vi "MTM2_putSample_ilcData.vi"(8 "error in (no error)":errorcluster, 11 "ilcData_Ctl":T1={"private_rcvStamp"=0.0, "status[78]"=[0, 0, 0, 0, 0, 0, 0, 0, 0, 0, 0, 0, 0, 0, 0, 0, 0, 0, 0, 0, 0, 0, 0, 0, 0, 0, 0, 0, 0, 0, 0, 0, 0, 0, 0, 0, 0, 0, 0, 0, 0, 0, 0, 0, 0, 0, 0, 0, 0, 0, 0, 0, 0, 0, 0, 0, 0, 0, 0, 0, 0, 0, 0, 0, 0, 0, 0, 0, 0, 0, 0, 0, 0, 0, 0, 0, 0, 0]}) -> (0 "error out":errorcluster, 2 "function return":i32, 3 "ilcData_Ctl out":T1)   [LabVIEW 2018, in "SALLV_MTM2.lvlib"]
doc: "int MTM2_shm_putSample_ilcDataLV(MTM2_ilcDataLV *ilcData_Ctl );"
uses:
  DataTypes/ilcData.ctl
  SALLV_MTM2.lvlib
  SALLV_MTM2.so
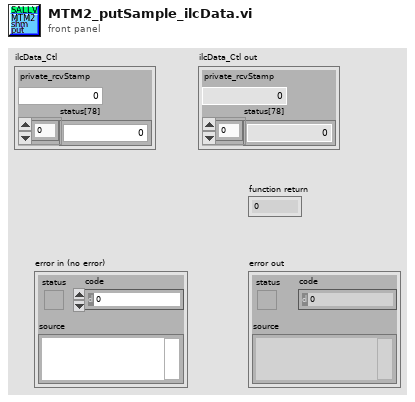
[diagram p1: front panel]
types:
  T1 = typedef "SALLV_MTM2.lvlib/ilcData.ctl" = cluster{"private_rcvStamp":dbl, "status[78]":u16[]}
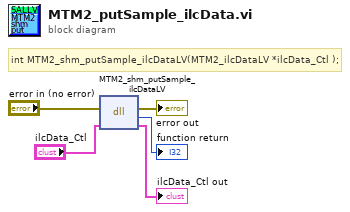
[diagram p0: block diagram]
diagram:
  # "int MTM2_shm_putSample_ilcDataLV(MTM2_ilcDataLV *ilcData_Ctl );"
  n1 = dll-call lib="home/ttsai/Documents/salLabviewApi/SALLV_MTM2/SALLV_MTM2.*" fn="MTM2_shm_putSample_ilcDataLV"(error in="error in (no error)", "ilcData_Ctl"="ilcData_Ctl") -> (error out=→"error out":errorcluster, →"function return":i32, "ilcData_Ctl"=→"ilcData_Ctl out":T1)  [unwired: 2 in, 1 out]
